vi "PythonPlotter.vi"(5 "Output File":string="C:\\Users\\TTUHEP\\Documents\\LabVIEW\\GantryPrograms\\LogFiles\\plot.png", 7 "error in (no error)":errorcluster, 8 "Function Name":string="plotter", 9 "Input File":string="C:\\Users\\TTUHEP\\Documents\\LabVIEW\\GantryPrograms\\Configs\\temp.txt", 10 "Python Path":path=path "C:/Users/TTUHEP/Documents/LabVIEW/GantryPrograms/Utilities/argParser.py") -> (0 "error out":errorcluster, 3 "HighVSPosition":picture)   [LabVIEW 2019]
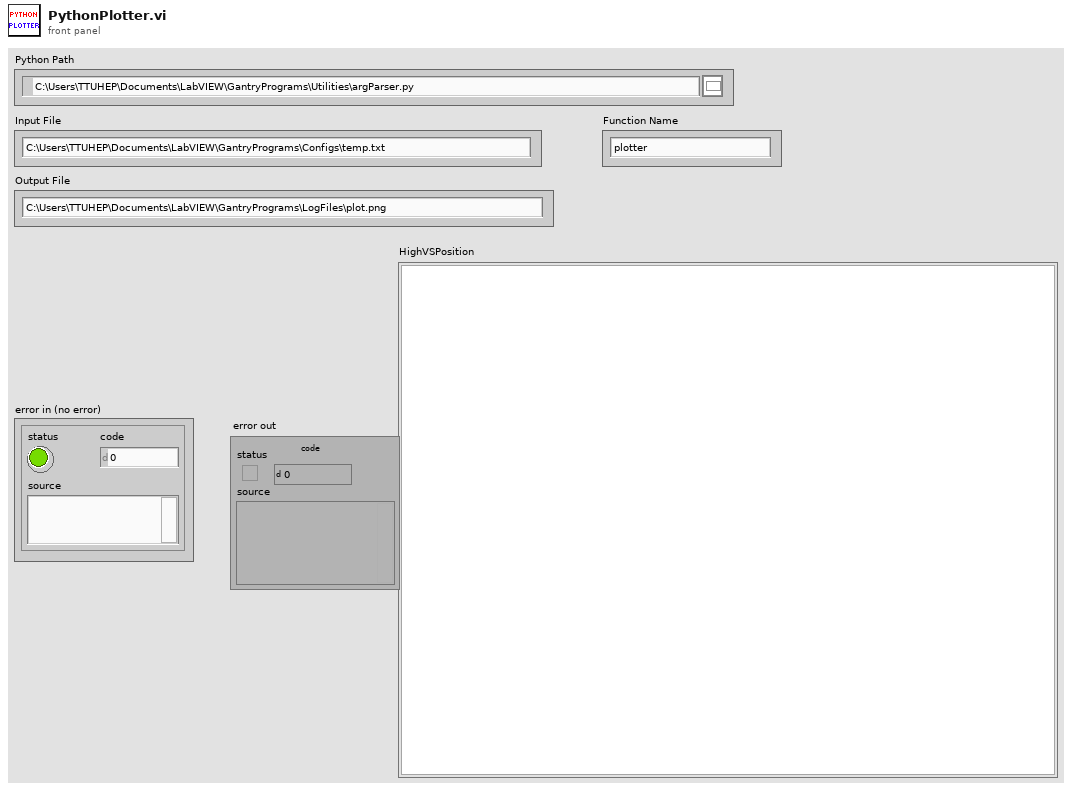
[diagram p1: front panel]
types:
  T1 = typedef "imagedata.ctl" = cluster{"image type":i32, "image depth":i32, "image":u8[], "mask":u8[], "colors":u32[], "Rectangle":cluster{"left":i16, "top":i16, "right":i16, "bottom":i16}}
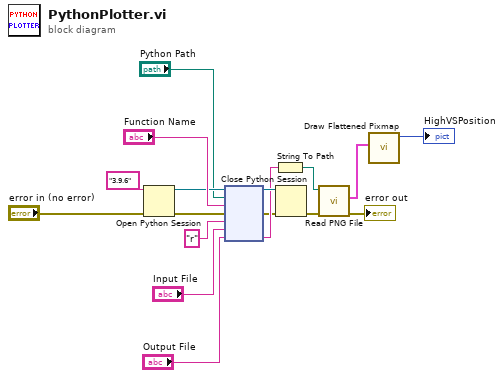
[diagram p0: block diagram]
diagram:
  n1 = Open Python Session(python version="3.9.6", 3:"error in (no error)") -> (session out=w15:refnum<k35>, error out=w4:errorcluster)  [unwired: 1 in]
  n2 = node(w15, "Python Path", "Function Name", w4, "r", "Input File", "Output File") -> (w10:refnum<k35>, w3:errorcluster, w9:string)  [unwired: 2 in, 2 out]
  n3 = String To Path(string=w9) -> (path=w8:path)
  n4 = Close Python Session(session in=w10, error in=w3) -> (11:w2:errorcluster)
  n5 = call <vilib>:"Read PNG File.vi"("error in (no error)"=w2, "path to PNG file"=w8) -> ("error out"=→"error out":errorcluster, "image data"=w7:T1)  [unwired: 7 in, 1 out]
  n6 = call <vilib>:"Draw Flattened Pixmap.vi"("image data"=w7) -> ("new picture"=→"HighVSPosition":picture)  [unwired: 8 in]
